vi "Initialize Attributes Core.vi"(8 "error in (no error)":errorcluster, 10 "Attribute Data":variant, 11 "BNT_ULx-MCSV-AIAvg in":refnum<class "BNT_ULx-MCSV-AIAvg.lvclass">) -> (0 "error out":errorcluster, 2 "MandatoryParameters":cluster{"Parameter":string, "found?":bool}[](array[cluster]), 3 "BNT_ULx-MCSV-AIAvg out":refnum<class "BNT_ULx-MCSV-AIAvg.lvclass">)   [LabVIEW 2020, in "BNT_ULx.lvlib" / "BNT_ULx-MCSV-AIAvg.lvclass"]
doc: "Initialize object attribute.\n\nUnique resources should be allocated elsewhere!"
uses:
  BNT_ULx-MCSV-AIAvg.lvclass
  BNT_ULx-MCSV-AIAvg.lvclass/BNT_ULx-MCSV-AIAvg.ctl
  BNT_ULx-MCSV/BNT_ULx-MCSV.lvclass
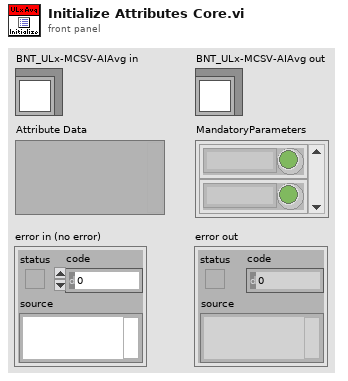
[diagram p1: front panel]
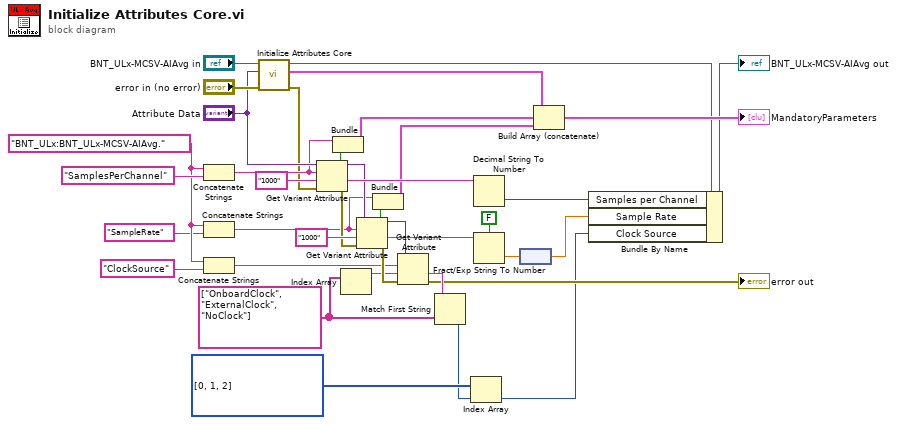
[diagram p0: block diagram]
diagram:
  w3 = i32[] [0, 1, 2] items=["OnboardClock", "ExternalClock", "NoClock"]
  w4 = string[] ["OnboardClock", "ExternalClock", "NoClock"]
  w17 = "BNT_ULx:BNT_ULx-MCSV-AIAvg."
  n1 = Concatenate Strings(w17, "SamplesPerChannel" ("string")) -> (w31:string)
  n2 = Concatenate Strings(w17, "SampleRate" ("string")) -> (w14:string)
  n3 = Concatenate Strings(w17, "ClockSource" ("string")) -> (w8:string)
  n4 = call-parent "Initialize Attributes Core.vi"("error in (no error)"="error in (no error)", "Attribute Data"="Attribute Data", "BNT_ULx-MCSV in"="BNT_ULx-MCSV-AIAvg in") -> ("error out"=w9:errorcluster, "MandatoryParameters"=w38:cluster{"Parameter":string, "found?":bool}[], "BNT_ULx-MCSV out"=w28:refnum<class "BNT_ULx-MCSV-AIAvg.lvclass">)  [unwired: 6 in]
  n5 = Get Variant Attribute(Variant="Attribute Data", name=w31, default value (empty Variant)="1000" ("string"), error in=w9) -> (duplicate Variant=w22:variant, found=w32:bool, value=w26:string, error out=w19:errorcluster)
  n6 = Bundle(w31, w32) -> (w29:cluster{string, bool})  [unwired: 1 in]
  n7 = Index Array(array=w4) -> (element=w5:string)  [unwired: 1 in]
  n8 = Get Variant Attribute(Variant=w22, name=w14, default value (empty Variant)="1000" ("string"), error in=w19) -> (duplicate Variant=w21:variant, found=w24:bool, value=w13:string, error out=w20:errorcluster)
  n9 = Bundle(w14, w24) -> (w18:cluster{string, bool})  [unwired: 1 in]
  n10 = Get Variant Attribute(Variant=w21, name=w8, default value (empty Variant)=w5, error in=w20) -> (value=w7:string, error out=→"error out":errorcluster)  [unwired: 2 out]
  n11 = Match First String(2:w4, 3:w7) -> (0:w2:i32)  [unwired: 1 out]
  n12 = Index Array(array=w3, index=w2) -> (element=w1:i32)
  n13 = Decimal String To Number(string=w26) -> (number=w25:i32)  [unwired: 2 in, 1 out]
  n14 = Fract/Exp String To Number(use system decimal point (T)=FALSE, string=w13) -> (number=w11:dbl)  [unwired: 2 in, 1 out]
  n15 = node(w11) -> (w10:dbl[unit])
  n16 = Build Array (concatenate)(w38, w29, w18) -> (→"MandatoryParameters":cluster{"Parameter":string, "found?":bool}[])
  n17 = Bundle By Name(cluster=w28, "Samples per Channel"=w25, "Sample Rate"=w10, "Clock Source"=w1) -> (→"BNT_ULx-MCSV-AIAvg out":refnum<class "BNT_ULx-MCSV-AIAvg.lvclass">)
